vi "Read Waveform (Multiple).vi"(8 "error in (no error)":errorcluster, 9 "Timeout (10000 ms)":u32=10000, 10 "Channels":u16[](array[ring])=[1, 2] items=["Channel 1"=1, "Channel 2"=2, "Channel 3"=3, "Channel 4"=4], 11 "VISA resource name":refnum<visa-resource-name>) -> (0 "error out":errorcluster, 2 "Waveform Data":waveform(dbl)[](graph), 3 "VISA resource name out":refnum<visa-resource-name>)   [LabVIEW 2021, in "Siglent SDS 1000 2000 Series.lvlib"]
doc: "Initiates an acquisition on all channels that you enabled with the <B>Configure Channel</B> VI. The VI waits for the acquisition to complete and returns the waveform for the Source Channels you specified. If the oscilloscope did not complete the acquisition within the time period you specify with the Timeout parameter, the VI returns a time out error. A common cause for a timeout error is the acquisition was not triggered. For example, the trigger level is out of range of the waveform. \n\nNote: If your instrument does not support auto compensation for probe attenuation, you may need to adjust the scaling of the Waveform Data accordingly. This is handled automatically in the <B>Configure Channel</B> VI or can be done manually by multiplying the Waveform Data by the probe attenuation."
uses:
  <instrlib>/Siglent SDS 1000 2000 Series/Siglent SDS 1000 2000 Series.lvlib
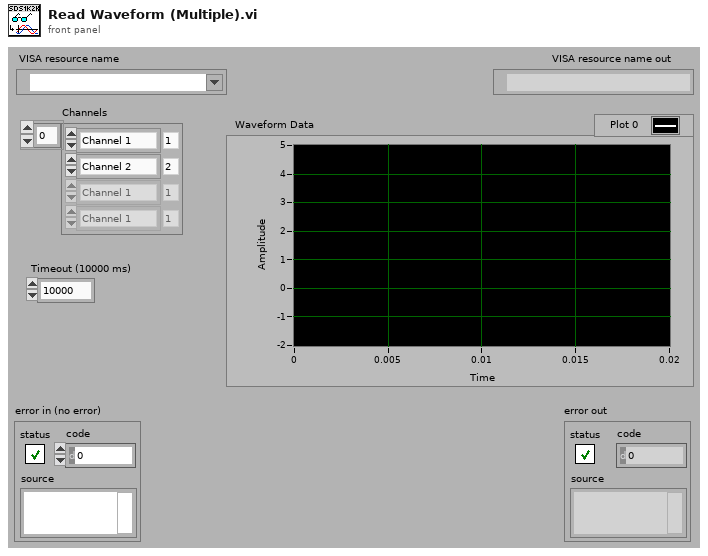
[diagram p1: front panel]
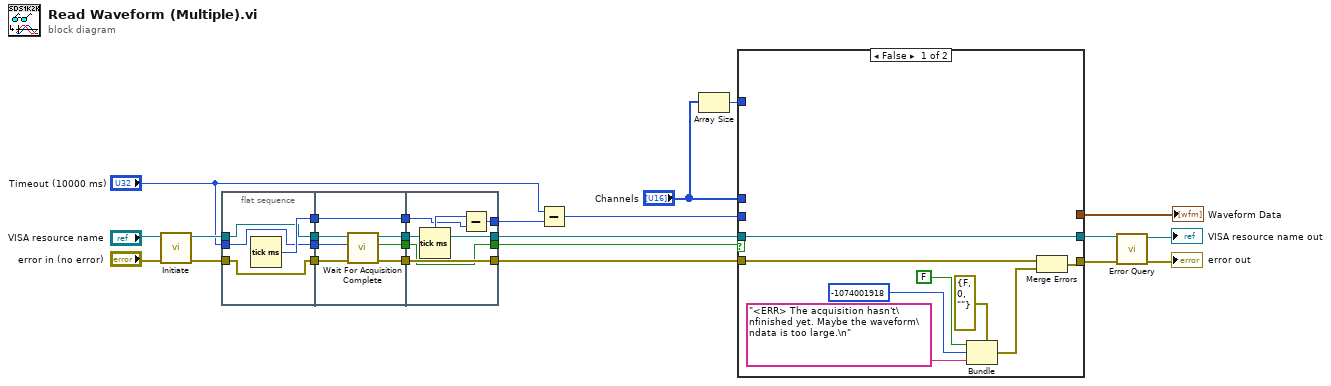
[diagram p0: block diagram]
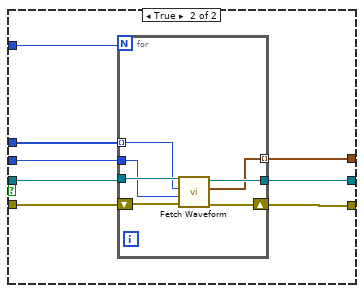
[diagram p2: hidden frame]
diagram:
  n1 = call <instrlib>:"Initiate.vi"("error in (no error)"="error in (no error)", "VISA resource name"="VISA resource name") -> ("error out"=w17:errorcluster, "VISA resource name out"=w18:refnum<visa-resource-name>)  [unwired: 8 in]
  n2 = flat-sequence {
    tunnel: "Timeout (10000 ms)" -> [w28]
    tunnel: [w28] -> w8
    tunnel: w18 -> [w27]
    tunnel: [w27] -> w7
    tunnel: w17 -> [w26]
    tunnel: [w26] -> w6
    tunnel: [w29] -> w5
    tunnel: w8 -> [w36]
    tunnel: w7 -> [w34]
    tunnel: w6 -> [w32]
    tunnel: [w31] -> w4
    tunnel: [w33] -> w3
    tunnel: [w35] -> w2
    tunnel: w5 -> [w30]
    tunnel: [w30] -> w1
    tunnel: [w39] -> w20
    tunnel: w4 -> [w39]
    tunnel: [w38] -> w21
    tunnel: w3 -> [w38]
    tunnel: [w40] -> w22
    tunnel: [w37] -> w19
    tunnel: w2 -> [w37]
    tunnel: w1 -> [w41]
    frame #0 {
      n3 = Tick Count (ms)() -> (millisecond timer value=w29:u32)
    }
    frame #1 {
      n4 = call <instrlib>:"Wait For Acquisition Complete.vi"("error in (no error)"=w32, "Timeout (10000 ms)"=w36, "VISA resource name"=w34) -> ("error out"=w31:errorcluster, "Complete"=w35:bool, "VISA resource name out"=w33:refnum<visa-resource-name>)  [unwired: 6 in]
    }
    frame #2 {
      n5 = Tick Count (ms)() -> (millisecond timer value=w42:u32)
      n6 = Subtract(x=w42, y=w41) -> (x-y=w40:u32)
    }
  }
  n7 = Subtract(x="Timeout (10000 ms)", y=w22) -> (x-y=w15:u32)
  n8 = Array Size(array="Channels") -> (size(s)=w9:i32)
  n9 = case shown="False" w19 {
    tunnel: [w50 w58] -> w14
    tunnel: [w44 w57] -> w13
    tunnel: [_ w56] -> w23
    tunnel: w21 -> [w50 w55]
    tunnel: w20 -> [w45 w54]
    tunnel: w15 -> [_ w53]
    tunnel: "Channels" -> [_ w52]
    tunnel: w9 -> [_ w51]
    frame False {
      n10 = Bundle(cluster=errorcluster {"status"=FALSE, "code"=0, "source"=""} ("error out"), "status"=FALSE, "code"=-1074001918 ("Code"), "source"="<ERR> The acquisition hasn't\nfinished yet. Maybe the waveform\ndata is too large.\n" ("Source")) -> (w46:errorcluster)
      n11 = Merge Errors(w45, w46) -> (w44:errorcluster)
    }
    frame True {
      n12 = for {
        N: w51 -> [_]
        tunnel: [w65] -> w58
        tunnel: w55 -> [w63]
        shift-right: [w64] -> w57
        shift-left: w54 -> [w62]
        tunnel: [w61] -> w56 mode=indexing
        tunnel: w53 -> [w59]
        tunnel: w52 -> [w60] mode=indexing
        n13 = call <instrlib>:"Fetch Waveform.vi"("error in (no error)"=w62, "Timeout (10000 ms)"=w59, "Source (1: Channel 1)"=w60, "VISA resource name"=w63) -> ("error out"=w64:errorcluster, "Waveform Graph"=w61:waveform(dbl), "VISA resource name out"=w65:refnum<visa-resource-name>)  [unwired: 5 in]
      }
    }
  }
  "Waveform Data" <- w23
  n14 = call <instrlib>:"Error Query.vi"("error in (no error)"=w13, "VISA resource name"=w14) -> ("error out"=→"error out":errorcluster, "VISA resource name out"=→"VISA resource name out":refnum<visa-resource-name>)  [unwired: 6 in, 2 out]
